vi "Substract Signals.vi"(0 "reference in":refnum<class "SigMath.lvclass">, 5 "error in (no error)":errorcluster, 7 "Sub Signals A":i32[](listbox) caption="Set A", 9 "Sub Signals B":i32[](listbox) caption="Set B") -> (14 "reference out":refnum<class "SigMath.lvclass">, 19 "error out":errorcluster)   [LabVIEW 2022 SP3, in "SigMath.lvclass"]
uses:
  SigMath.lvclass
  API/GSwFormDSP_class/functions/Attribute List.ctl
  API/GSwFormDSP_class/functions/Attribute Options.ctl
  API/GSwFormDSP_class/GSwFormDSP.lvclass
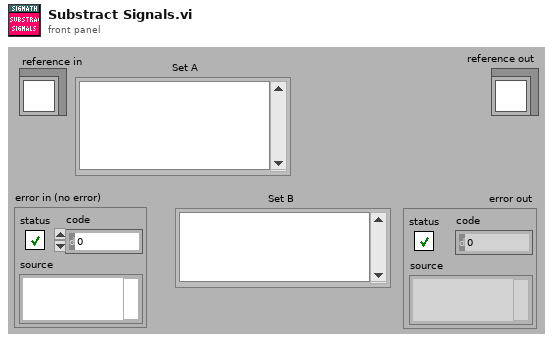
[diagram p1: front panel]
types:
  T1 = typedef "GSwFormDSP.lvclass/Attribute Options.ctl" = enum16{"Append to Attribute using \"( )\"", "Replace Attribute Value"}
  T2 = typedef "GSwFormDSP.lvclass/Attribute List.ctl" = string
  T3 = typedef "SigMath.lvclass/ObjectAttributes.ctl" = cluster{"SigMath Data":T4, "User CTRL Refs":T5}
  T4 = typedef "SigMath.lvclass/SigMath Data.ctl" = cluster{"New Time Data Obj?":bool, "GSwFormDSP":refnum<class "GSwFormDSP.lvclass">}
  T5 = typedef "SigMath.lvclass/SigMath User CTRL Refs.ctl" = cluster{"wForms":refnum<vi>, "Results wForms":refnum<vi>}
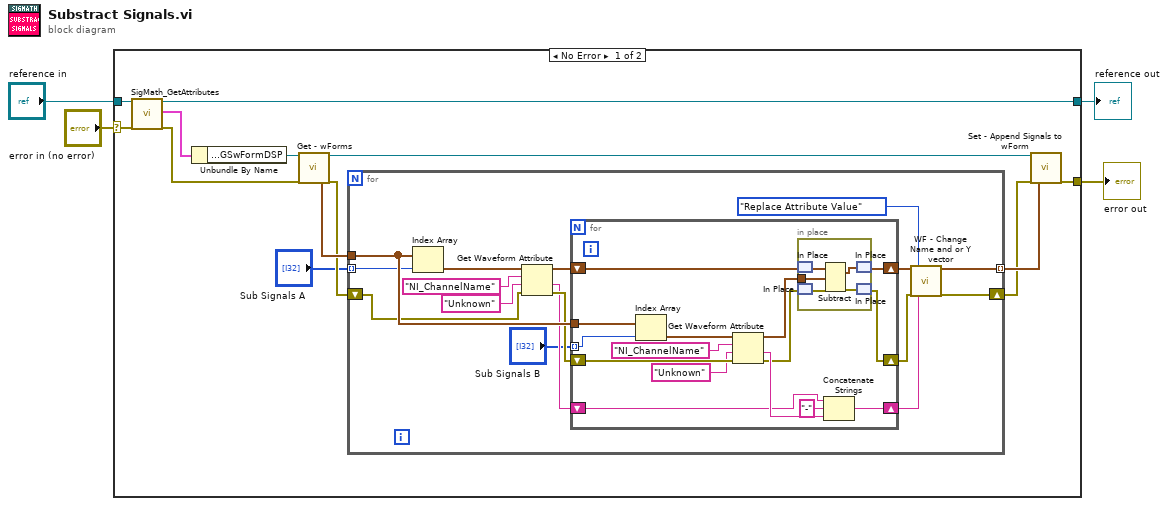
[diagram p0: block diagram]
diagram:
  n1 = case shown="No Error" "error in (no error)" {
    selector: "error in (no error)" -> [w17 w55]
    tunnel: [w10 w55] -> w3
    tunnel: [w16 w54] -> w1
    tunnel: "reference in" -> [w15 w54]
    frame No Error {
      n2 = call "SigMath_GetAttributes.vi"("reference in"=w15, "error in (no error)"=w17) -> ("reference out"=w16:refnum<class "SigMath.lvclass">, "attributes"=w14:T3, "error out"=w12:errorcluster)  [unwired: 14 in, 1 out]
      n3 = Unbundle By Name(w14) -> ("SigMath Data.GSwFormDSP"=w11:refnum<class "GSwFormDSP.lvclass">)
      n4 = call-dynamic "Get - wForms.vi"("reference in"=w11, "error in (no error)"=w12) -> ("wForms"=w13:waveform(dbl)[], "reference out"=w9:refnum<class "GSwFormDSP.lvclass">, "error out"=w7:errorcluster)  [unwired: 14 in, 1 out]
      n5 = for {
        tunnel: w13 -> [w33]
        tunnel: [w20] -> w8 mode=indexing
        shift-right: [w21] -> w6
        shift-left: w7 -> [w28]
        tunnel: "Sub Signals A" -> [w19] mode=indexing
        n6 = Index Array(array=w33, index=w19) -> (element=w31:waveform(dbl))
        n7 = Get Waveform Attribute(4:w28, 5:"Unknown", 6:T2 "NI_ChannelName" ("Attribute List"), 7:w31) -> (0:w27:errorcluster, 1:w26:string, 3:w30:waveform(dbl))  [unwired: 1 out]
        n8 = for {
          shift-right: [w38] -> w25
          shift-left: w30 -> [w39]
          tunnel: w33 -> [w48]
          shift-right: [w35] -> w23
          shift-left: w27 -> [w46]
          shift-right: [w40] -> w22
          shift-left: w26 -> [w41]
          tunnel: "Sub Signals B" -> [w34] mode=indexing
          n9 = Index Array(array=w48, index=w34) -> (element=w47:waveform(dbl))
          n10 = Get Waveform Attribute(4:w46, 5:"Unknown", 6:T2 "NI_ChannelName" ("Attribute List"), 7:w47) -> (0:w36:errorcluster, 1:w42:string, 3:w37:waveform(dbl))  [unwired: 1 out]
          n11 = in-place {
            in-place-border: w37 -> [w52]
            n12 = in-place-match #1(w39) -> (w53:waveform(dbl))
            n13 = in-place-match #2(w36) -> (w51:errorcluster)
            n14 = Subtract(1:w52, 2:w53, 4:w51) -> (0:w50:waveform(dbl), 3:w49:errorcluster)
            n15 = in-place-match #1(w50) -> (w38:waveform(dbl))
            n16 = in-place-match #2(w49) -> (w35:errorcluster)
          }
          n17 = Concatenate Strings(w41, "-" ("string"), w42) -> (w40:string)
        }
        n18 = call "WF - Change Name and or Y vector.vi"("wForm IN"=w25, "error in (no error)"=w23, "Attribute Option"=Attribute_Options."Replace Attribute Value", "SigName Update"=w22) -> ("wForm OUT"=w20:waveform(dbl), "error out"=w21:errorcluster)  [unwired: 14 in]
      }
      n19 = call "Set - Append Signals to wForm.vi"("reference in"=w9, "error in (no error)"=w6, "New Signals"=w8) -> ("error out"=w10:errorcluster)  [unwired: 15 in, 1 out]
    }
    frame Error {
    }
  }
  "error out" <- w3
  "reference out" <- w1
